vi "Read Sum.vi"(0 "TwinCAT ADS in":refnum<class "TwinCAT ADS.lvclass">, 5 ".NET Type Stream":refnum<k24>[](array[refnum]), 9 "Handles":u32[](array[numeric]), 11 "error in (no error)":errorcluster) -> (4 "TwinCAT ADS out":refnum<class "TwinCAT ADS.lvclass">, 8 ".NET Object Stream":refnum<k24>[](array[refnum]), 10 "Handles":u32[](array[numeric]), 15 "error out":errorcluster)   [LabVIEW 2018, in "TwinCAT ADS.lvclass"]
uses:
  TwinCAT ADS.lvclass
  TwinCAT.Ads
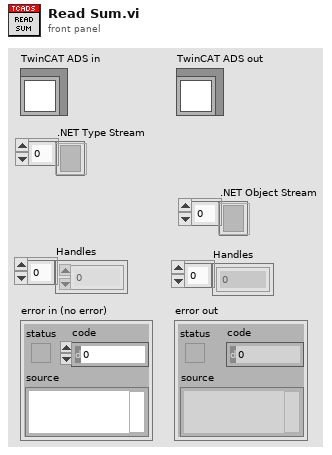
[diagram p1: front panel]
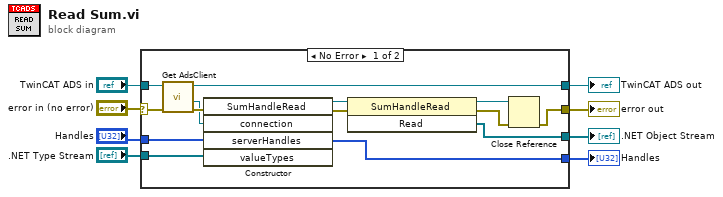
[diagram p0: block diagram]
diagram:
  n1 = case shown="No Error" "error in (no error)" {
    selector: "error in (no error)" -> [w21 w24]
    tunnel: [w19 w24] -> w7
    tunnel: [w20 w23] -> w5
    tunnel: "TwinCAT ADS in" -> [w22 w23]
    tunnel: "Handles" -> [w14 _]
    tunnel: ".NET Type Stream" -> [w13 _]
    tunnel: [w12 _] -> w2
    tunnel: [w9 _] -> w1
    frame No Error {
      n2 = call-dynamic "Get AdsClient.vi"("error in (no error)"=w21, "TwinCAT ADS in"=w22) -> ("error out"=w16:errorcluster, ".NET TcAdsClient refnum"=w11:refnum<k24>, "TwinCAT ADS out"=w20:refnum<class "TwinCAT ADS.lvclass">)  [unwired: 7 in]
      n3 = constructor class="SumHandleRead"(error in=w16, "connection"=w11, "serverHandles"=w14, "valueTypes"=w13) -> (reference out=w17:refnum<k24>, error out=w18:errorcluster, "serverHandles"=w9:u32[])  [unwired: 2 in, 3 out]
      n4 = invoke class="SumHandleRead" method="Read"(reference=w17, error in=w18) -> (reference out=w10:refnum<k24>, error out=w15:errorcluster, "Read"=w12:refnum<k24>[])  [unwired: 1 in]
      n5 = Close Reference(reference=w10, error in (no error)=w15) -> (error out=w19:errorcluster)
    }
    frame Error {
    }
  }
  "error out" <- w7
  "TwinCAT ADS out" <- w5
  ".NET Object Stream" <- w2
  "Handles" <- w1
